vi "hw2subvi.vi"(7 "Voltage":dbl(slide) scale=0.0..4.0 scale format="%#.3f", 8 "Unit Selector":u16(ring) items=["Celsius", "Fahrenheit", "Kelvin"]) -> (0 "Temperature":dbl(slide) scale=-350.0..600.0 scale format="%#.3g", 1 "Units":string, 2 "Input too low":bool, 3 "Input too high":bool)   [LabVIEW 2011]
uses:
  <vilib>/express/express arith-compare/Formula/XNode/ExpressFormulaBlockNode.xnode
panel:
  out "Invalid Range Danger":bool
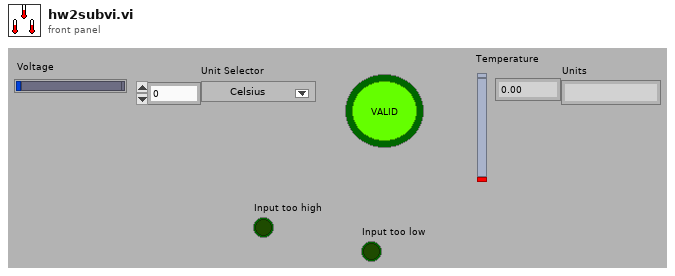
[diagram p1: front panel]
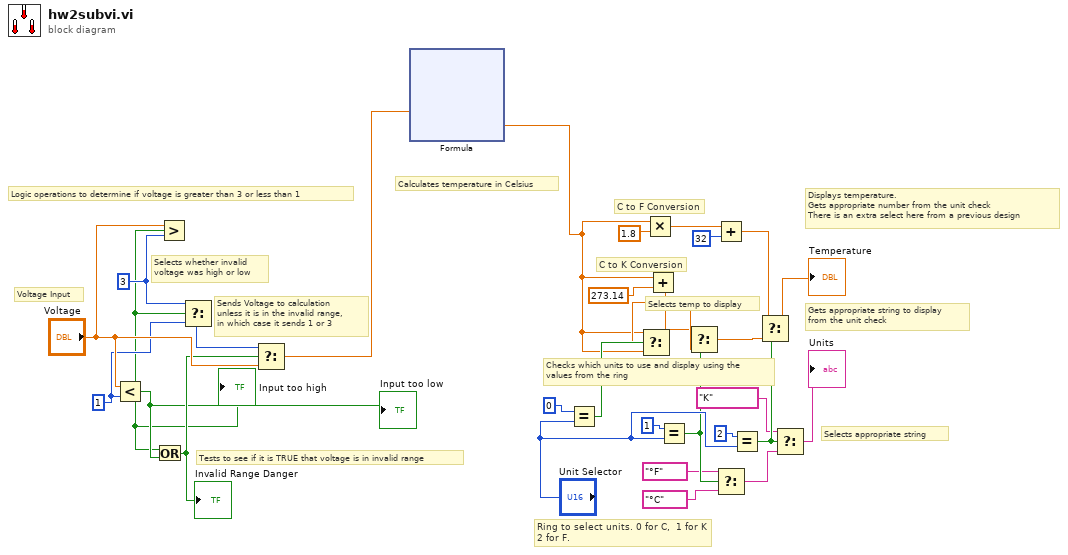
[diagram p0: block diagram]
diagram:
  w27 = 3
  w26 = 1
  # "Selects temp to display"
  # "C to F Conversion"
  # "C to K Conversion"
  # "Selects appropriate string"
  # "Displays temperature. \nGets appropriate number from the unit check \nThere is an extra select here from a previous design"
  # "Gets appropriate string to display\nfrom the unit check"
  # "Checks which units to use and display using the\nvalues from the ring"
  # "Ring to select units. 0 for C,  1 for K\n2 for F."
  # "Calculates temperature in Celsius"
  # "Selects whether invalid \nvoltage was high or low"
  # "Sends Voltage to calculation\nunless it is in the invalid range, \nin which case it sends 1 or 3"
  # "Tests to see if it is TRUE that voltage is in invalid range"
  # "Logic operations to determine if voltage is greater than 3 or less than 1"
  # "Voltage Input"
  n1 = Less?(x="Voltage", y=w26) -> (x < y?=w4:bool)
  "Input too low" <- w4
  n2 = Greater?(x="Voltage", y=w27) -> (0:w3:bool)
  "Input too high" <- w3
  n3 = Or(x=w3, y=w4) -> (x .or. y?=w29:bool)
  "Invalid Range Danger" <- w29
  n4 = Select(t=w27, s=w3, f=w26) -> (s? t:f=w28:i32)
  n5 = Select(t=w28, s=w29, f="Voltage") -> (s? t:f=w2:dbl)
  n6 = xnode "Formula"("X1"=w2) -> ("Result"=w1:dbl)  [unwired: 1 in, 1 out]
  n7 = Equal?(x=0, y="Unit Selector") -> (x = y?=w22:bool)
  n8 = Select(t=w1, s=w22, f=w1) -> (s? t:f=w16:dbl)
  n9 = Multiply(x=w1, y=1.8) -> (x*y=w18:dbl)
  n10 = Add(x=w1, y=273.14) -> (x+y=w15:dbl)
  n11 = Equal?(x=1, y="Unit Selector") -> (x = y?=w12:bool)
  n12 = Select(t=w15, s=w12, f=w16) -> (s? t:f=w14:dbl)
  n13 = Add(x=w18, y=32) -> (x+y=w13:dbl)
  n14 = Select(t="°F", s=w12, f="°C") -> (s? t:f=w9:string)
  n15 = Equal?(x=2, y="Unit Selector") -> (x = y?=w8:bool)
  n16 = Select(t=w13, s=w8, f=w14) -> (s? t:f=→"Temperature":dbl)
  n17 = Select(t="K", s=w8, f=w9) -> (s? t:f=→"Units":string)
